vi "RDB Receive Core.vi"(6 "index":i32, 7 "paeseHandle in":u64, 8 "error in (no error)":errorcluster, 9 "RDB Data in":T1[](array[typedef]) {"payload" format="%x"; "timestamp" format="%<%.7X\n%x>T"; "type" items=["FlexRay Data"=32, "FlexRay Null"=33, "FlexRay Symbol"=34, "Log Trigger"=225, "Start Trigger"=226]; "cycle count" max=63 step=1}, 10 "vclient":path, 11 "XNET Conversion":refnum<k21>) -> (0 "error out":errorcluster, 2 "signal data":dbl[](array[numeric]), 3 "RDB Data out":T1[](array[typedef]) {"payload" format="%x"; "timestamp" format="%<%.7X\n%x>T"; "type" items=["FlexRay Data"=32, "FlexRay Null"=33, "FlexRay Symbol"=34, "Log Trigger"=225, "Start Trigger"=226]; "cycle count" max=63 step=1})   [LabVIEW 2023, in "RDB.lvlib"]
uses:
  RDB.lvlib
  <vilib>/xnet/xnet.llb/XNET Frame FlexRay.ctl
  <vilib>/xnet/xnet.llb/XNET Frame Type FlexRay.ctl
  <vilib>/xnet/xnet.llb/XNET Convert (Frame FlexRay to Signal).vi
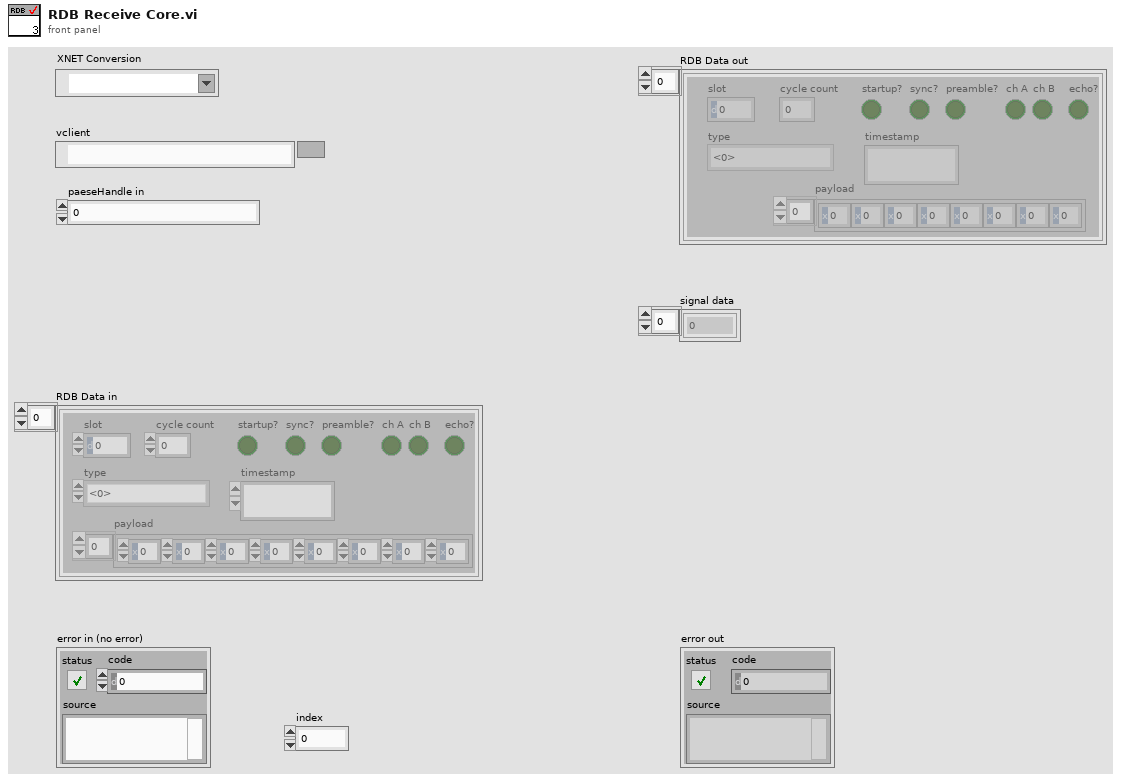
[diagram p1: front panel]
types:
  T1 = typedef "XNET Frame FlexRay.ctl" = cluster{"timestamp":timestamp, "payload":u8[], "slot":u16, "type":T2, "cycle count":u8, "startup?":bool, "sync?":bool, "preamble?":bool, "ch A":bool, "ch B":bool, "echo?":bool}
  T2 = typedef "XNET Frame Type FlexRay.ctl" = u8
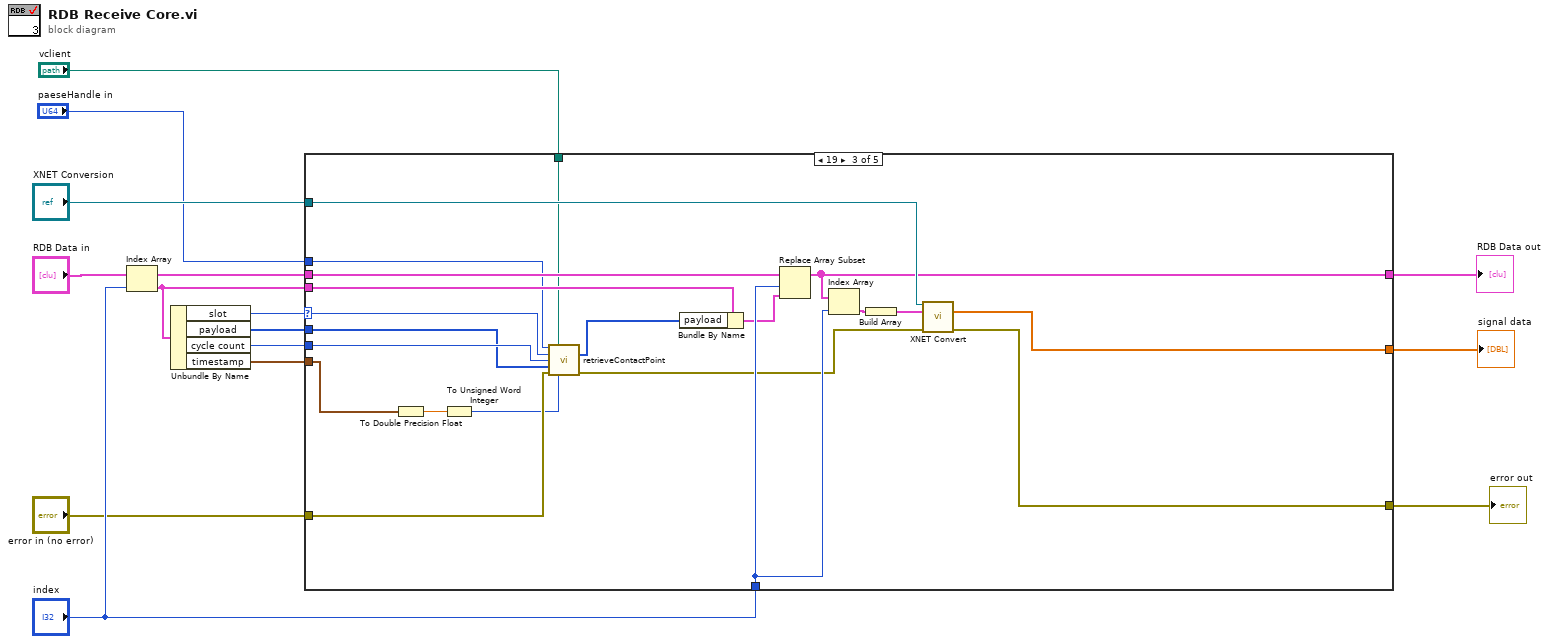
[diagram p0: block diagram]
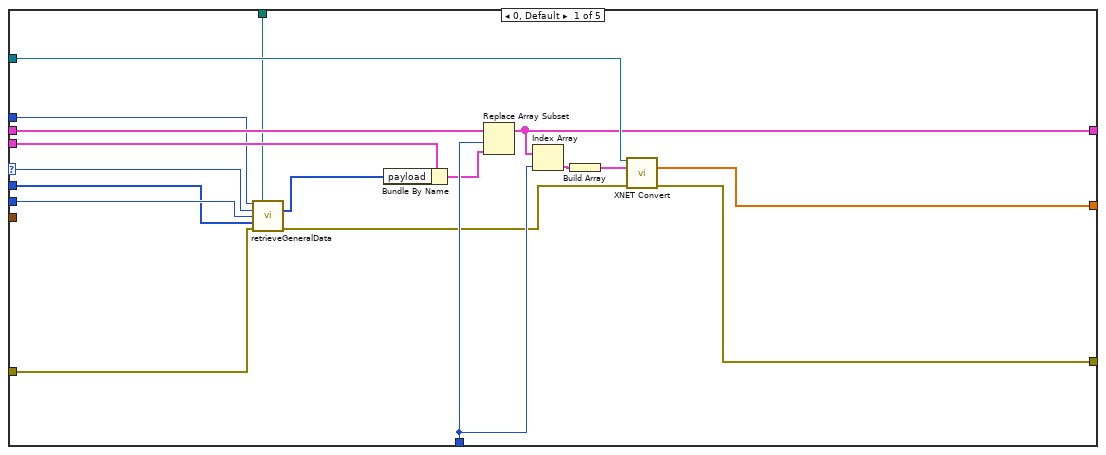
[diagram p2: hidden frame]
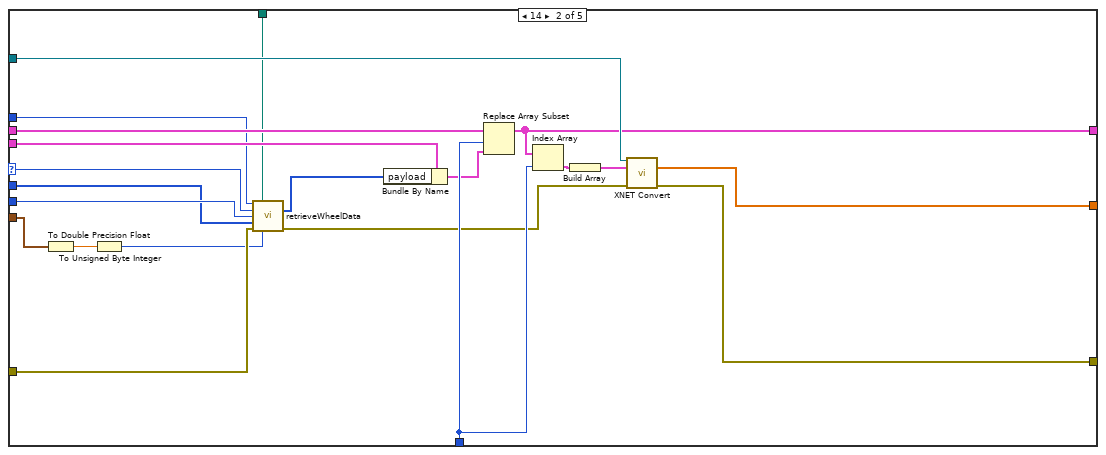
[diagram p3: hidden frame]
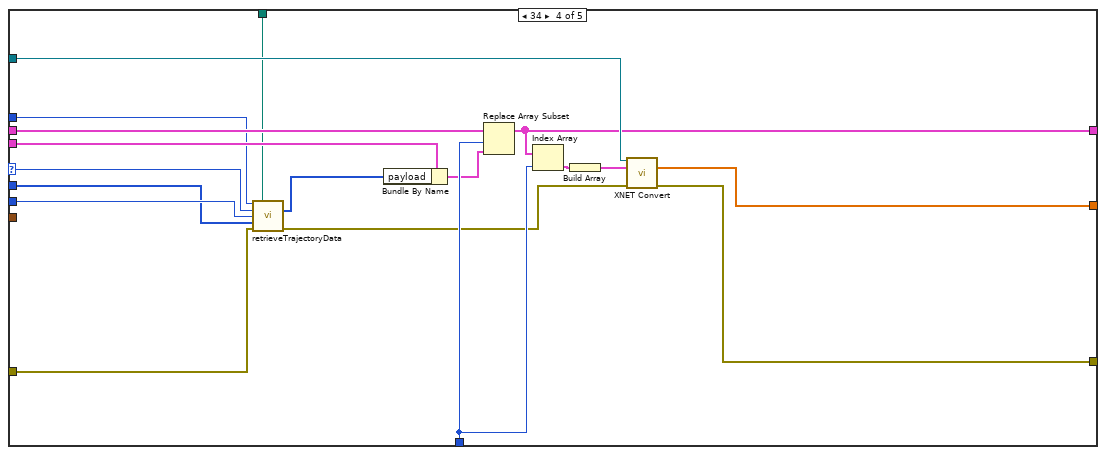
[diagram p4: hidden frame]
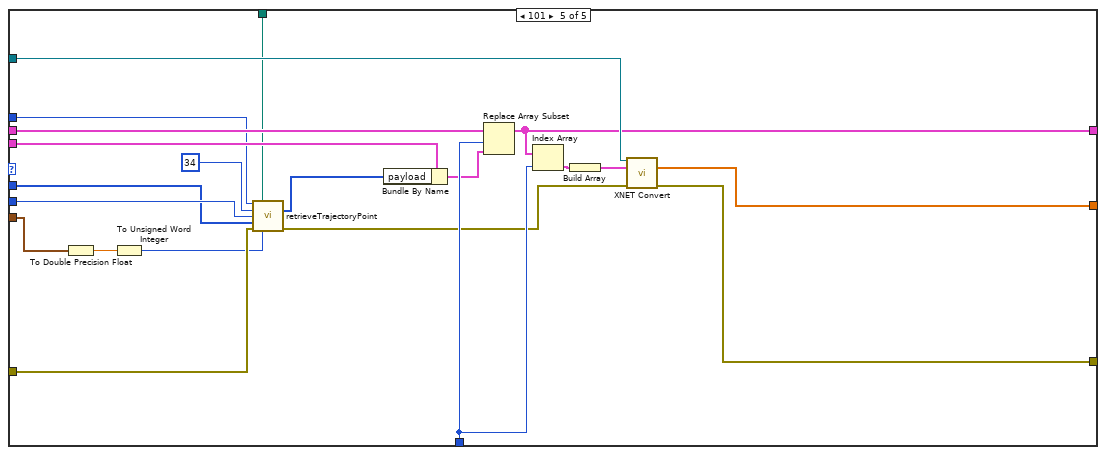
[diagram p5: hidden frame]
diagram:
  n1 = Index Array(array="RDB Data in", index="index") -> (element=w5:T1)
  n2 = Unbundle By Name(w5) -> ("slot"=w2:u16, "payload"=w14:u8[], "cycle count"=w4:u8, "timestamp"=w13:timestamp)
  n3 = case shown="19" w2 {
    selector: w2 -> [w17 w38 w57 w77 _]
    tunnel: w14 -> [w15 w33 w58 w75 w97]
    tunnel: w13 -> [_ w36 w55 _ w94]
    tunnel: "vclient" -> [w22 w43 w64 w82 w103]
    tunnel: [w32 w53 w74 w92 w113] -> w11
    tunnel: [w31 w52 w73 w91 w112] -> w10
    tunnel: "XNET Conversion" -> [w29 w50 w71 w89 w110]
    tunnel: "index" -> [w27 w48 w69 w87 w108]
    tunnel: [w26 w47 w68 w86 w107] -> w7
    tunnel: "RDB Data in" -> [w24 w45 w66 w84 w105]
    tunnel: w5 -> [w23 w44 w65 w83 w104]
    tunnel: w4 -> [w16 w37 w59 w76 w98]
    tunnel: "error in (no error)" -> [w21 w42 w63 w81 w102]
    tunnel: "paeseHandle in" -> [w18 w39 w60 w78 w99]
    frame 0, Default {
      n4 = call "retrieveGeneralData.vi"("paeseHandle in"=w18, "path in"=w22, "packageID"=w17, "playerID"=w16, "dataOut"=w15, "error in (no error)"=w21) -> ("dataOut"=w19:u8[], "error out"=w20:errorcluster)  [unwired: 7 in, 1 out]
      n5 = Bundle By Name(cluster=w23, "payload"=w19) -> (w25:T1)
      n6 = Replace Array Subset(array=w24, new element=w25, index=w27) -> (w26:T1[])
      n7 = Index Array(array=w26, index=w27) -> (element=w28:T1)
      n8 = Build Array(w28) -> (w30:T1[])
      n9 = call-poly <vilib>:"XNET Convert.vi"("session in"=w29, "frame data"=w30, "error in (no error)"=w20) -> ("signal data"=w32:dbl[], "error out"=w31:errorcluster)  [unwired: 10 in, 1 out]
    }
    frame 14 {
      n10 = To Double Precision Float(number=w36) -> (double precision float=w34:dbl)
      n11 = To Unsigned Byte Integer(number=w34) -> (unsigned 8bit integer=w35:u8)
      n12 = call "retrieveWheelData.vi"("paeseHandle in"=w39, "path in"=w43, "packageID"=w38, "playerID"=w37, "dataOut"=w33, "error in (no error)"=w42, "wheelID"=w35) -> ("dataOut"=w40:u8[], "error out"=w41:errorcluster)  [unwired: 6 in, 1 out]
      n13 = Bundle By Name(cluster=w44, "payload"=w40) -> (w46:T1)
      n14 = Replace Array Subset(array=w45, new element=w46, index=w48) -> (w47:T1[])
      n15 = Index Array(array=w47, index=w48) -> (element=w49:T1)
      n16 = Build Array(w49) -> (w51:T1[])
      n17 = call-poly <vilib>:"XNET Convert.vi"("session in"=w50, "frame data"=w51, "error in (no error)"=w41) -> ("signal data"=w53:dbl[], "error out"=w52:errorcluster)  [unwired: 10 in, 1 out]
    }
    frame 19 {
      n18 = To Double Precision Float(number=w55) -> (double precision float=w56:dbl)
      n19 = To Unsigned Word Integer(number=w56) -> (unsigned 16bit integer=w54:u16)
      n20 = call "retrieveContactPoint.vi"("paeseHandle in"=w60, "path in"=w64, "packageID"=w57, "playerID"=w59, "dataOut"=w58, "error in (no error)"=w63, "pointID"=w54) -> ("dataOut"=w61:u8[], "error out"=w62:errorcluster)  [unwired: 6 in, 1 out]
      n21 = Bundle By Name(cluster=w65, "payload"=w61) -> (w67:T1)
      n22 = Replace Array Subset(array=w66, new element=w67, index=w69) -> (w68:T1[])
      n23 = Index Array(array=w68, index=w69) -> (element=w70:T1)
      n24 = Build Array(w70) -> (w72:T1[])
      n25 = call-poly <vilib>:"XNET Convert.vi"("session in"=w71, "frame data"=w72, "error in (no error)"=w62) -> ("signal data"=w74:dbl[], "error out"=w73:errorcluster)  [unwired: 10 in, 1 out]
    }
    frame 34 {
      n26 = call "retrieveTrajectoryData.vi"("paeseHandle in"=w78, "path in"=w82, "packageID"=w77, "playerID"=w76, "dataOut"=w75, "error in (no error)"=w81) -> ("dataOut"=w79:u8[], "error out"=w80:errorcluster)  [unwired: 7 in, 1 out]
      n27 = Bundle By Name(cluster=w83, "payload"=w79) -> (w85:T1)
      n28 = Replace Array Subset(array=w84, new element=w85, index=w87) -> (w86:T1[])
      n29 = Index Array(array=w86, index=w87) -> (element=w88:T1)
      n30 = Build Array(w88) -> (w90:T1[])
      n31 = call-poly <vilib>:"XNET Convert.vi"("session in"=w89, "frame data"=w90, "error in (no error)"=w80) -> ("signal data"=w92:dbl[], "error out"=w91:errorcluster)  [unwired: 10 in, 1 out]
    }
    frame 101 {
      n32 = To Double Precision Float(number=w94) -> (double precision float=w96:dbl)
      n33 = To Unsigned Word Integer(number=w96) -> (unsigned 16bit integer=w95:u16)
      n34 = call "retrieveTrajectoryPoint.vi"("paeseHandle in"=w99, "path in"=w103, "packageID"=u16 34, "playerID"=w98, "dataOut"=w97, "error in (no error)"=w102, "pointIndex"=w95) -> ("dataOut"=w100:u8[], "error out"=w101:errorcluster)  [unwired: 6 in, 1 out]
      n35 = Bundle By Name(cluster=w104, "payload"=w100) -> (w106:T1)
      n36 = Replace Array Subset(array=w105, new element=w106, index=w108) -> (w107:T1[])
      n37 = Index Array(array=w107, index=w108) -> (element=w109:T1)
      n38 = Build Array(w109) -> (w111:T1[])
      n39 = call-poly <vilib>:"XNET Convert.vi"("session in"=w110, "frame data"=w111, "error in (no error)"=w101) -> ("signal data"=w113:dbl[], "error out"=w112:errorcluster)  [unwired: 10 in, 1 out]
    }
  }
  "signal data" <- w11
  "error out" <- w10
  "RDB Data out" <- w7
